vi "Update Tag String.vi"(8 "error in (no error)":errorcluster, 9 "string":string caption="String", 10 "Tag Path":string, 11 "Logger in.lvclass":refnum<class "Logger.lvclass">) -> (0 "error out":errorcluster, 3 "Logger out.lvclass":refnum<class "Logger.lvclass">)   [LabVIEW 2016, in "Logger.lvclass"]
uses:
  Logger.lvclass
  Logger.lvclass/Logger.ctl
  <vilib>/TagLibrary/Generate Tag Cluster (String).vi
  <vilib>/TagLibrary/TagLibrary.lvlib
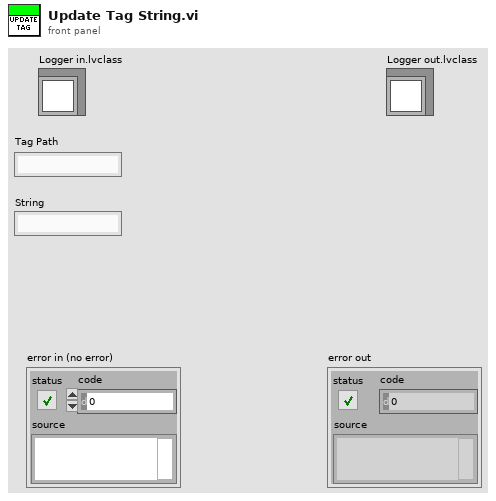
[diagram p1: front panel]
types:
  T1 = cluster{"Tag Reference":refnum<k21>, "Tag Units":string, "Tag Path":string, "Waveform":waveform(dbl), "Log":bool}[]
  T2 = typedef "TagLibrary.lvlib/TagCluster.ctl" = cluster{"tag reference":refnum<k21>, "value":variant, "timestamp":timestamp, "data type":T3}
  T3 = typedef "TagLibrary.lvlib/DataType.ctl" = enum32{"Double", "Integer", "String"}
  T4 = cluster{"Tag Reference":refnum<k21>, "Tag Units":string, "Tag Path":string, "Waveform":waveform(dbl), "Log":bool}
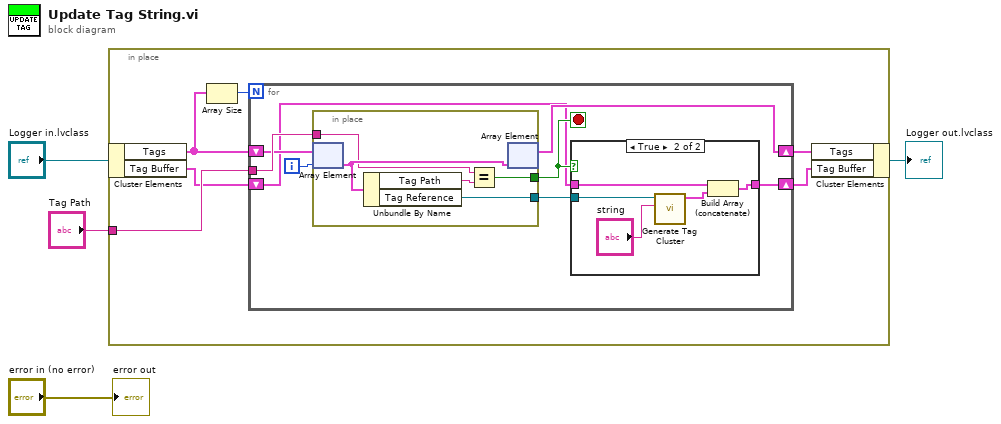
[diagram p0: block diagram]
diagram:
  n1 = in-place {
    in-place-border: "Tag Path" -> [w10]
    n2 = in-place-cluster #1("Logger in.lvclass") -> ("Tags"=w7:T1, "Tag Buffer"=w6:T2[])
    n3 = Array Size(array=w7) -> (size(s)=w8:i32)
    n4 = for {
      N: w8 -> [_]
      tunnel: w10 -> [w18]
      shift-right: [w13] -> w9
      shift-left: w7 -> [w17]
      shift-right: [w11] -> w5
      shift-left: w6 -> [w12]
      i -> [w16]
      stop <- w15 stop-if-true
      n5 = in-place {
        in-place-border: w18 -> [w26]
        in-place-border: [w27] -> w15
        in-place-border: [w29] -> w14
        n6 = in-place-array #2(w17, w16) -> (w28:T4)
        n7 = Unbundle By Name(w28) -> ("Tag Path"=w25:string, "Tag Reference"=w29:refnum<k21>)
        n8 = Equal?(x=w26, y=w25) -> (x = y?=w27:bool)
        n9 = in-place-array #2(w28) -> (w13:T1)  [unwired: 1 out]
      }
      n10 = case shown="True" w15 {
        tunnel: w14 -> [_ w24]
        tunnel: w12 -> [w19 w22]
        tunnel: [w19 w21] -> w11
        frame False {
        }
        frame True {
          n11 = call-poly <vilib>:"Generate Tag Cluster.vi"("string"="string", "tag reference in"=w24) -> ("tag cluster"=w20:T2)  [unwired: 9 in]
          n12 = Build Array (concatenate)(w22, w20) -> (w21:T2[])
        }
      }
    }
    n13 = in-place-cluster #1("Tags"=w9, "Tag Buffer"=w5) -> (→"Logger out.lvclass":refnum<class "Logger.lvclass">)
  }
  "error out" <- "error in (no error)"
